vi "Teleop.vi"(10 "Match Info":T1={"Autonomous Elapsed Seconds"=0.0, "TeleOp Elapsed Seconds"=0.0, "Disabled Elapsed Seconds"=0.0, "Visited Autonomous"=FALSE, "Visited TeleOp"=FALSE, "Visited Disabled"=FALSE, "Autonomous Settings"={"Autonomous Style"=enum."Independent", "VI Refnum"=refnum}}, 11 "Call Context":T2) -> ()   [LabVIEW 2013]
doc: "This VI is called for each TeleOp packet received from the DS where the robot is not disabled. It is often used to read from the joysticks and update I/O or to update setpoints for timed control loops. It should complete and return within 20 milliseconds or it may miss DS packets."
uses:
  <vilib>/Rock Robotics/WPI/DriverStation/WPI_DriverStationDerivedRobotMode.ctl
  <vilib>/Rock Robotics/WPI/DriverStation/WPI_DriverStationMatch Info.ctl
  <vilib>/Rock Robotics/WPI/Solenoid/WPI_SolenoidValue.ctl
  Robot Global Data.vi
  Device Refrences.vi
  <vilib>/Rock Robotics/WPI/Solenoid/WPI_SolenoidSetEnum.vi
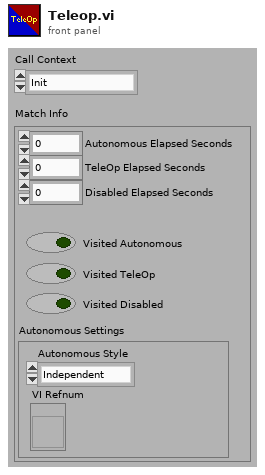
[diagram p1: front panel]
types:
  T1 = typedef "WPI_DriverStationMatch Info.ctl" = cluster{"Autonomous Elapsed Seconds":dbl, "TeleOp Elapsed Seconds":dbl, "Disabled Elapsed Seconds":dbl, "Visited Autonomous":bool, "Visited TeleOp":bool, "Visited Disabled":bool, "Autonomous Settings":cluster{"Autonomous Style":enum16{"Iterative", "Independent"}, "VI Refnum":refnum<vi>}}
  T2 = typedef "WPI_DriverStationDerivedRobotMode.ctl" = enum16{"Init", "Execute", "Stop"}
  T3 = typedef "WPI_SolenoidValue.ctl" = enum16{"Off", "On", "Forward", "Reverse"}
  T4 = cluster{"Shooter":cluster{"Shoot Ball":bool, "Short Range":bool, "Long Range":bool, "Retract Shooter":bool, "Running shot":bool, "Low goal shot":bool}, "Drive":cluster{"Drive Y":dbl, "Drive X":dbl, "Speed Throttle":bool}, "Pickup":cluster{"Pickup Motor":dbl, "Extend Pickup":bool, "Retract Pickup":bool, "Eject Ball":bool}}
  T5 = cluster{"Compressor running":bool, "Compressor enabled":bool, "Right Encoder":dbl, "Left Encoder":dbl, "Ultrasonic Sensor":dbl, "Light Sensor":dbl, "Gyro":dbl, "Left Encoder Speed":dbl, "Ball Presence":bool, "Pressure":dbl}
  T6 = typedef "WPI_RobotDriveDevRef.ctl" = cluster{"DevStatus":errorcluster, "Motors[]":T7[], "Square Inputs":bool, "Max Output":dbl, "Isochronous":bool}
  T7 = typedef "WPI_MotorControlDeviceRef.ctl" = cluster{"DeviceStatus":errorcluster, "Type":enum16{"PWM", "CAN"}, "PWM":cluster{"Digital Module":T8, "PWM Channel":T9, "DeadBand":T10}, "CAN":cluster{"Device Number":u8, "Control Mode":T11, "Semaphore":T12, "Max Vout":dbl}, "Invert":bool, "TransformRef":T13, "InvTransformRef":T13}
  T8 = typedef "FPGA_TypedefDigitalModule.ctl" = enum16{"Digital Module 1", "Digital Module 2"}
  T9 = typedef "FPGA_DIOPWMChannel.ctl" = enum8{"PWM 1", "PWM 2", "PWM 3", "PWM 4", "PWM 5", "PWM 6", "PWM 7", "PWM 8", "PWM 9", "PWM 10", "Invalid"}
  T10 = typedef "WPI_PWMDeadband.ctl" = cluster{"Name":string, "maxPositivePwm":i32, "minPositivePwm":i32, "centerPwm":i32, "maxNegativePwm":i32, "minNegativePwm":i32, "angularRange":u16}
  T11 = typedef "WPI_CANJaguar_ControlMode.ctl" = enum8{"Percent VBus", "Current", "Speed", "Position", "Voltage"}
  T12 = typedef "Semaphore RefNum" = refnum<k1>
  T13 = typedef "WPI_PWMTransform_ConPane.ctl" = refnum<vi>
  T14 = cluster{"Drive Output Values":dbl[], "Shooter Solenoid":T3, "Pickup Solenoid":T3, "Pickup Motor":dbl, "Ejecter Solenoid":T3}
  T15 = enum16{"Simulator Robot", "Alpinista", "2014 Robot"}
  T16 = typedef "WPI_SolenoidDevRef.ctl" = cluster{"DevStatus":errorcluster, "Solenoid Module":T17, "Forward Solenoid Channel":T18, "Reverse Solenoid Channel":T18}
  T17 = typedef "FPGA_TypedefSolenoidModule.ctl" = enum16{"Solenoid Module 1", "Solenoid Module 2"}
  T18 = typedef "WPI_SolenoidChannel.ctl" = enum8{"Solenoid 1", "Solenoid 2", "Solenoid 3", "Solenoid 4", "Solenoid 5", "Solenoid 6", "Solenoid 7", "Solenoid 8", "Invalid"}
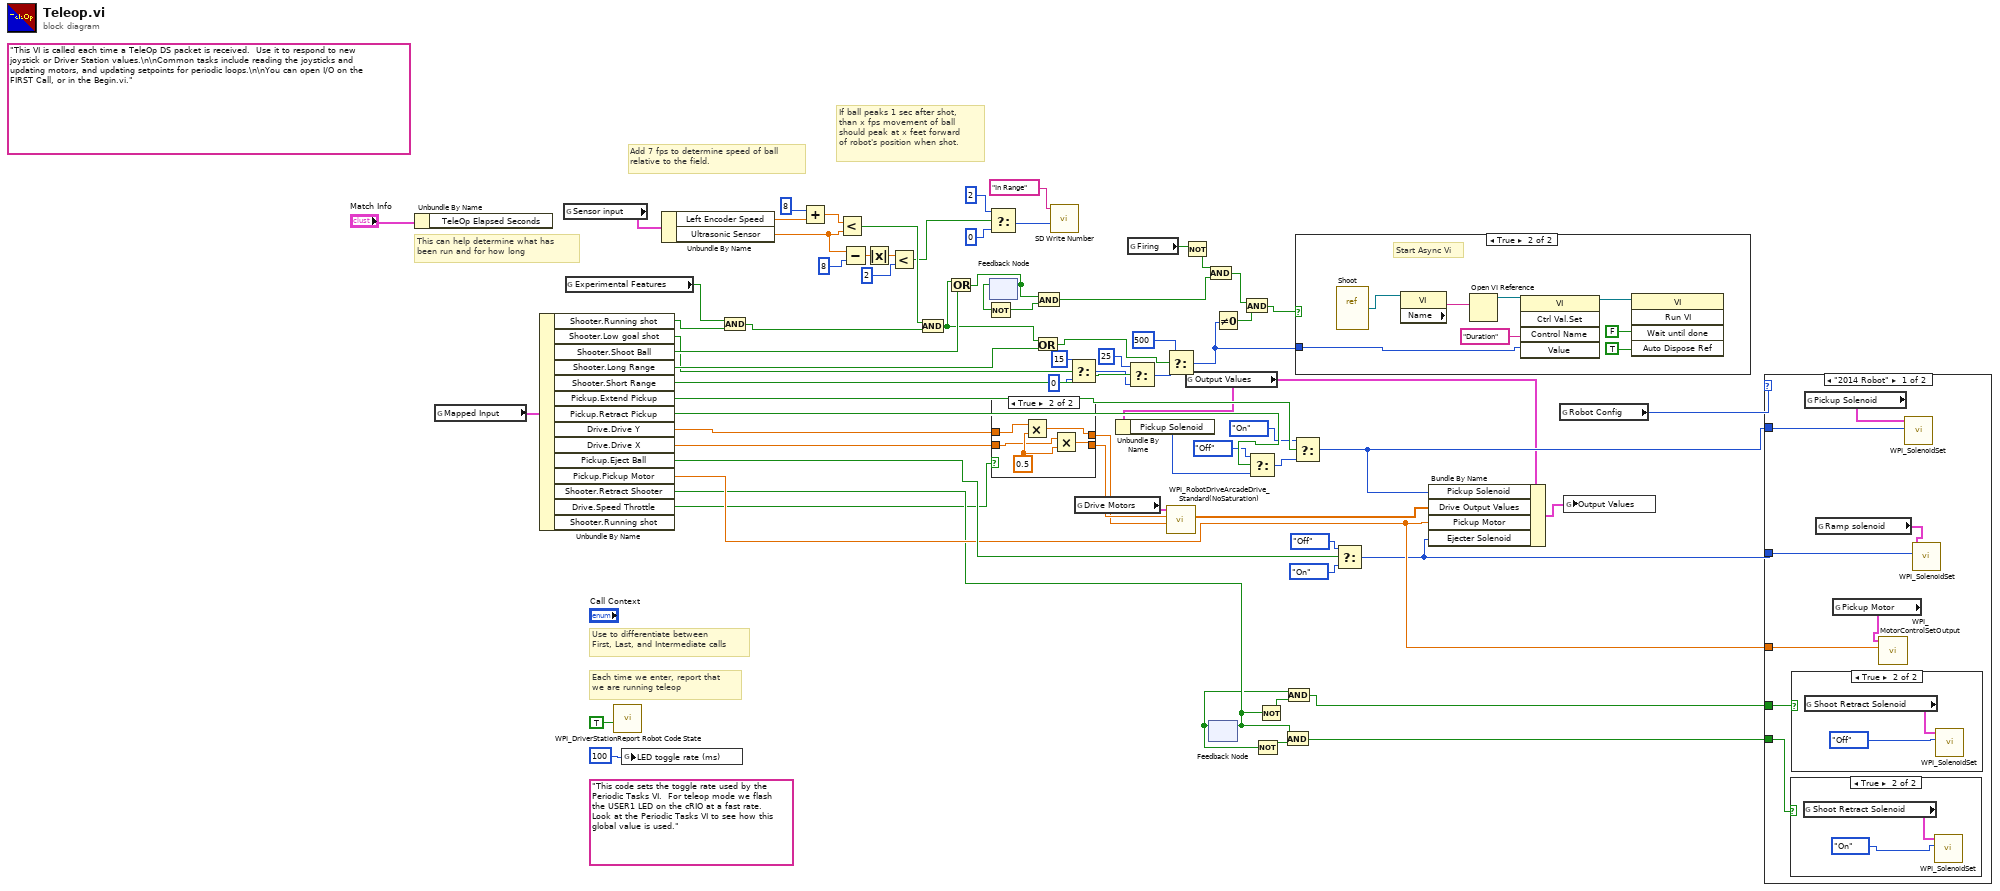
[diagram p0: block diagram]
diagram:
  (unwired) "This code sets the toggle rate used by the Periodic Tasks VI.  For teleop mode we flash the USER1 LED on the cRIO at a fast rate.  Look at the Periodic Tasks VI to see how this global value is used."
  (unwired) "This VI is called each time a TeleOp DS packet is received.  Use it to respond to new joystick or Driver Station values.\n\nCommon tasks include reading the joysticks and updating motors, and updating setpoints for periodic loops.\n\nYou can open I/O on the FIRST Call, or in the Begin.vi."
  # "If ball peaks 1 sec after shot,\nthan x fps movement of ball\nshould peak at x feet forward\nof robot's position when shot."
  # "Add 7 fps to determine speed of ball\nrelative to the field."
  # "Each time we enter, report that\nwe are running teleop"
  # "Use to differentiate between\nFirst, Last, and Intermediate calls"
  # "This can help determine what has\nbeen run and for how long"
  n1 = Unbundle By Name("Match Info") -> ()  [unwired: 1 out]
  n2 = global read "Robot Global Data.vi" "Mapped Input"() -> (w68:T4)
  n3 = Unbundle By Name(w68) -> ("Shooter.Running shot"=w25:bool, "Shooter.Low goal shot"=w19:bool, "Shooter.Shoot Ball"=w28:bool, "Shooter.Long Range"=w29:bool, "Shooter.Short Range"=w61:bool, "Pickup.Extend Pickup"=w62:bool, "Pickup.Retract Pickup"=w63:bool, "Drive.Drive Y"=w36:dbl, "Drive.Drive X"=w38:dbl, "Pickup.Eject Ball"=w58:bool, "Pickup.Pickup Motor"=w55:dbl, "Shooter.Retract Shooter"=w45:bool, "Drive.Speed Throttle"=w39:bool)  [unwired: 1 out]
  n4 = global read "Robot Global Data.vi" "Sensor input"() -> (w15:T5)
  n5 = global read "Robot Global Data.vi" "Experimental Features"() -> (w26:bool)
  n6 = call <vilib>:"WPI_DriverStationReport Robot Code State.vi"("TeleOp"=TRUE ("Autonomous")) -> ()  [unwired: 10 in, 1 out]
  n7 = global write "Robot Global Data.vi" "LED toggle rate (ms)"(u32 100 ("LED ms toggle rate")) -> ()
  n8 = Unbundle By Name(w15) -> ("Left Encoder Speed"=w17:dbl, "Ultrasonic Sensor"=w5:dbl)
  n9 = And(x=w26, y=w25) -> (x .and. y?=w10:bool)
  n10 = Add(x=8, y=w17) -> (x+y=w6:dbl)
  n11 = Less?(x=w6, y=w5) -> (x < y?=w4:bool)
  n12 = Subtract(x=w5, y=8) -> (x-y=w7:dbl)
  n13 = Absolute Value(x=w7) -> (abs(x)=w3:dbl)
  n14 = Less?(x=w3, y=2) -> (x < y?=w1:bool)
  n15 = And(x=w4, y=w10) -> (x .and. y?=w9:bool)
  n16 = Or(x=w9, y=w28) -> (x .or. y?=w27:bool)
  n17 = Select(t=2, s=w1, f=0) -> (s? t:f=w12:i32)
  n18 = feedback-in #1(w27) -> ()
  n19 = feedback #1() -> (w32:bool)  [unwired: 1 in]
  n20 = Not(x=w32) -> (.not. x?=w31:bool)
  n21 = case shown="True" w39 {
    tunnel: w38 -> [w73 w75]
    tunnel: [w73 w79] -> w37
    tunnel: w36 -> [w74 w76]
    tunnel: [w74 w77] -> w35
    frame False {
    }
    frame True {
      w78 = 0.5
      n22 = Multiply(x=w76, y=w78) -> (x*y=w77:dbl)
      n23 = Multiply(x=w75, y=w78) -> (x*y=w79:dbl)
    }
  }
  n24 = Or(x=w9, y=w29) -> (x .or. y?=w22:bool)
  n25 = And(x=w27, y=w31) -> (x .and. y?=w30:bool)
  n26 = call <vilib>:"SD Write Number.vi"("Numeric"=w12, "Name"="In Range") -> ()  [unwired: 8 in, 2 out]
  n27 = Select(t=15, s=w19, f=0) -> (s? t:f=w20:i32)
  n28 = global read "Device Refrences.vi" "Drive Motors"() -> (w69:T6)
  n29 = global read "Robot Global Data.vi" "Firing"() -> (w60:bool)
  n30 = Select(t=25, s=w61, f=w20) -> (s? t:f=w46:i32)
  n31 = Select(t=500, s=w22, f=w46) -> (s? t:f=w24:i32)
  n32 = call <vilib>:"WPI_RobotDriveArcadeDrive_Standard(NoSaturation).vi"("Y axis value"=w35, "X axis value"=w37, "RobotDriveDevRef"=w69) -> ("Motor Values"=w66:dbl[])  [unwired: 1 in, 7 out]
  n33 = Not(x=w60) -> (.not. x?=w59:bool)
  n34 = global read "Robot Global Data.vi" "Output Values"() -> (w34:T14)
  n35 = Unbundle By Name(w34) -> ("Pickup Solenoid"=w33:T3)
  n36 = And(x=w59, y=w30) -> (x .and. y?=w48:bool)
  n37 = feedback-in #2(w45) -> ()
  n38 = feedback #2() -> (w43:bool)  [unwired: 1 in]
  n39 = Not Equal To 0?(x=w24) -> (x != 0?=w49:bool)
  n40 = And(x=w48, y=w49) -> (x .and. y?=w50:bool)
  n41 = Select(t=WPI_SolenoidValue."Off" ("Value"), s=w63, f=w33) -> (s? t:f=w64:T3)
  n42 = Not(x=w43) -> (.not. x?=w44:bool)
  n43 = Not(x=w45) -> (.not. x?=w42:bool)
  n44 = And(x=w45, y=w44) -> (x .and. y?=w41:bool)
  n45 = And(x=w43, y=w42) -> (x .and. y?=w40:bool)
  n46 = Select(t=WPI_SolenoidValue."On" ("Value"), s=w62, f=w64) -> (s? t:f=w54:T3)
  n47 = case shown="True" w50 {
    tunnel: w24 -> [_ w80]
    frame False {
    }
    frame True {
      # "Start Async Vi"
      n48 = vi-ref "Shoot.vi"() -> (w86:refnum<vi>)
      n49 = property class="VI"(reference=w86) -> ("Name"=w87:string)  [unwired: 1 in, 2 out]
      n50 = Open VI Reference(vi path=w87) -> (vi reference=w85:refnum<vi>)  [unwired: 2 in, 4 out]
      n51 = invoke class="VI" method="Ctrl Val.Set"(reference=w85, "Control Name"="Duration", "Value"=w80) -> (reference out=w83:refnum<vi>)  [unwired: 2 in, 4 out]
      n52 = invoke class="VI" method="Run VI"(reference=w83, "Wait until done"=FALSE, "Auto Dispose Ref"=TRUE) -> ()  [unwired: 2 in, 5 out]
    }
  }
  n53 = Select(t=WPI_SolenoidValue."Off" ("Value"), s=w58, f=WPI_SolenoidValue."On" ("Value")) -> (s? t:f=w51:T3)
  n54 = Bundle By Name(cluster=w34, "Pickup Solenoid"=w54, "Drive Output Values"=w66, "Pickup Motor"=w55, "Ejecter Solenoid"=w51) -> (w65:T14)
  n55 = global read "Robot Global Data.vi" "Robot Config"() -> (w67:T15)
  n56 = global write "Robot Global Data.vi" "Output Values"(w65) -> ()
  n57 = case shown="\"2014 Robot\"" w67 {
    tunnel: w54 -> [w94 _]
    tunnel: w51 -> [w92 _]
    tunnel: w55 -> [w90 _]
    tunnel: w41 -> [w89 _]
    tunnel: w40 -> [w88 _]
    frame "2014 Robot" {
      n58 = case shown="True" w89 {
        frame False {
        }
        frame True {
          n59 = global read "Device Refrences.vi" "Shoot Retract Solenoid"() -> (w97:T16)
          n60 = call-poly <vilib>:"WPI_SolenoidSet.vi"("Value"=WPI_SolenoidValue."On", "SolenoidDevRef"=w97) -> ()  [unwired: 8 in, 2 out]
        }
      }
      n61 = case shown="True" w88 {
        frame False {
        }
        frame True {
          n62 = global read "Device Refrences.vi" "Shoot Retract Solenoid"() -> (w99:T16)
          n63 = call-poly <vilib>:"WPI_SolenoidSet.vi"("Value"=WPI_SolenoidValue."Off", "SolenoidDevRef"=w99) -> ()  [unwired: 8 in, 2 out]
        }
      }
      n64 = global read "Device Refrences.vi" "Pickup Solenoid"() -> (w95:T16)
      n65 = global read "Device Refrences.vi" "Ramp solenoid"() -> (w93:T16)
      n66 = global read "Device Refrences.vi" "Pickup Motor"() -> (w91:T7)
      n67 = call <vilib>:"WPI_MotorControlSetOutput.vi"("Output"=w90, "MotorControlDevRef"=w91) -> ()  [unwired: 7 in, 3 out]
      n68 = call-poly <vilib>:"WPI_SolenoidSet.vi"("Value"=w94, "SolenoidDevRef"=w95) -> ()  [unwired: 8 in, 2 out]
      n69 = call-poly <vilib>:"WPI_SolenoidSet.vi"("Value"=w92, "SolenoidDevRef"=w93) -> ()  [unwired: 8 in, 2 out]
    }
    frame "Simulator Robot", Default {
    }
  }
